vi "Global RPM simulati.vi"() -> ()   [LabVIEW 2019]
panel:
  out "Rpm simulati":dbl
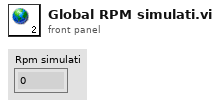
[diagram p1: front panel]
diagram:
